vi "ResetFlowMeter.vi"(8 "error in (no error)":errorcluster, 11 "Queue in":refnum<queue>) -> (0 "error out 2":errorcluster)   [LabVIEW 2020]
uses:
  Message Queue/Message Cluster.ctl
  Message Queue/Enqueue Message (Single).vi
  Message Queue/Message Queue.lvlib
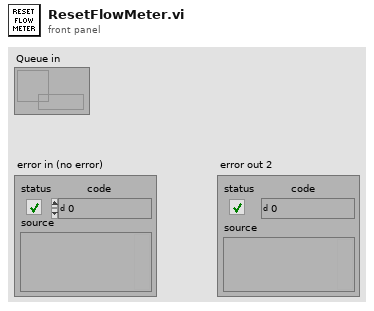
[diagram p1: front panel]
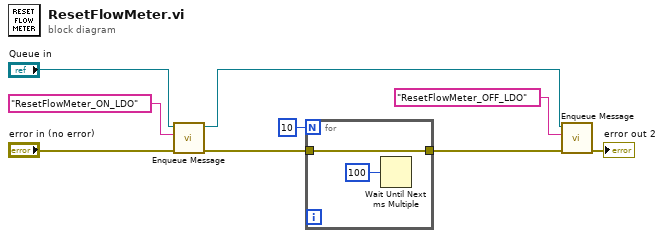
[diagram p0: block diagram]
diagram:
  n1 = call-poly "Enqueue Message.vi"("error in (no error)"="error in (no error)", "Message"="ResetFlowMeter_ON_LDO", "Message Queue"="Queue in") -> ("error out"=w8:errorcluster, "dup Message Queue"=w3:refnum<queue>)  [unwired: 7 in]
  n2 = for {
    N: 10 -> [_]
    tunnel: w8 -> [w10]
    tunnel: [w10] -> w9
    n3 = Wait Until Next ms Multiple(millisecond multiple=u32 100) -> ()  [unwired: 1 out]
  }
  n4 = call-poly "Enqueue Message.vi"("error in (no error)"=w9, "Message"="ResetFlowMeter_OFF_LDO", "Message Queue"=w3) -> ("error out"=→"error out 2":errorcluster)  [unwired: 7 in, 1 out]
